vi "SubVI TX Add Freq Offset.vi"(8 "samples per symbol":i32, 9 "frequency offset":dbl, 10 "symbol rate (Hz)":dbl=100000000.0 format="%#_6p", 11 "输入":cdb[](array[numeric])) -> (3 "输出":cdb[](array[numeric]))   [LabVIEW 2015]
uses:
  <vilib>/Analysis/1siggen.llb/Ramp Pattern by Samples.vi
  <vilib>/Analysis/NI_AALBase.lvlib
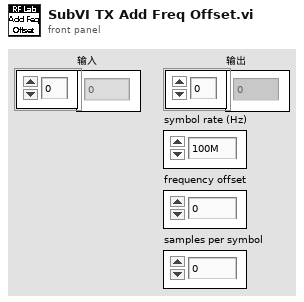
[diagram p1: front panel]
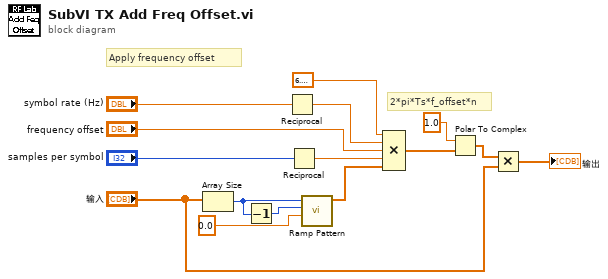
[diagram p0: block diagram]
diagram:
  # "Apply frequency offset"
  # "2*pi*Ts*f_offset*n"
  n1 = Array Size(array="输入") -> (size(s)=w13:i32)
  n2 = Decrement(x=w13) -> (x-1=w14:i32)
  n3 = Reciprocal(x="symbol rate (Hz)") -> (1/x=w7:dbl)
  n4 = Reciprocal(x="samples per symbol") -> (1/x=w6:dbl)
  n5 = call-poly <vilib>:"Ramp Pattern.vi"("start"=0.0, "end"=w14, "samples"=w13) -> ("Ramp Pattern"=w11:dbl[])  [unwired: 7 in, 1 out]
  n6 = Compound Arithmetic op=MULTIPLY(6.283185307179586, w7, "frequency offset", w6, w11) -> (w9:dbl[])
  n7 = Polar To Complex(1:w9, 2:1.0 ("r")) -> (0:w8:cdb[])
  n8 = Multiply(x=w8, y="输入") -> (x*y=→"输出":cdb[])
